vi "test_list.vi"   [LabVIEW 2020]
uses:
  g_ar_toolkit/g_ar_toolkit.32.dll
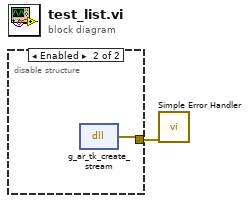
[diagram p0: block diagram]
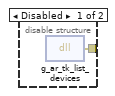
[diagram p2: hidden frame]
diagram:
  n1 = disable-structure shown="Enabled" {
    disable-tunnel: [w2 w3] -> w1
    frame Disabled {
      n2 = dll-call lib="C:/serenial/libraries/g-augmented-reality-toolkit/LabVIEW/g_ar_toolkit/g_ar_toolkit.32.dll" fn="g_ar_tk_list_devices"() -> (error out=w2:errorcluster)  [unwired: 4 in, 1 out]
    }
    frame Enabled {
      n3 = dll-call lib="C:/serenial/libraries/g-augmented-reality-toolkit/LabVIEW/g_ar_toolkit/g_ar_toolkit.32.dll" fn="g_ar_tk_create_stream"() -> (error out=w3:errorcluster)  [unwired: 4 in, 1 out]
    }
  }
  n4 = call <vilib>:"Simple Error Handler.vi"("error in (no error)"=w1) -> ()  [unwired: 4 in, 5 out]
